vi "configure.vi"(8 "error in (no error)":errorcluster, 10 "SerialConfig":T1={"Serial Protocol"=enum."RS485", "Protocol Parameters"={"VISA resource name"="", "Baud Rate"=9600, "Data Bits"=8, "Parity"=enum."None", "Flow Control"=0, "Stop Bits"=10, "Timeout (ms)"=10000}} {"Protocol Parameters"."Stop Bits" items=["1.0"=10, "1.5"=15, "2.0"=20]; "Protocol Parameters"."Flow Control" items=["None", "XON/XOFF", "RTS/CTS", "XON/XOFF & RTS/CTS", "DTR/DSR", "XON/XOFF & DTR/DSR"]; "Protocol Parameters"."Data Bits" min=5 max=8 step=1}, 11 "SerialCommunicator in":refnum<class "SerialCommunicator.lvclass">) -> (0 "error out":errorcluster, 3 "SerialCommunicator out":refnum<class "SerialCommunicator.lvclass">)   [LabVIEW 2013, in "SerialProtocols.lvlib" / "SerialCommunicator.lvclass"]
uses:
  <userlib>/Common/SerialProtocols/SerialCommunicator/SerialCommunicator.lvclass
  <userlib>/Common/SerialProtocols/Configuration/SerialConfig.ctl
  <userlib>/Common/SerialProtocols/Configuration/SerialProtocol.ctl
  <userlib>/Common/SerialProtocols/Configuration/ProtocolParameters.ctl
  <userlib>/Common/SerialProtocols/SerialCommunicator/SerialCommunicator.lvclass/SerialCommunicator.ctl
  <userlib>/Common/SerialProtocols/SerialProtocolFactory/ISerialProtocolFactory/ISerialProtocolFactory.lvclass
  <userlib>/Common/SerialProtocols/SerialProtocol/SerialProtocol/SerialProtocol.lvclass
  <userlib>/Common/SerialProtocols/SerialProtocols.lvlib
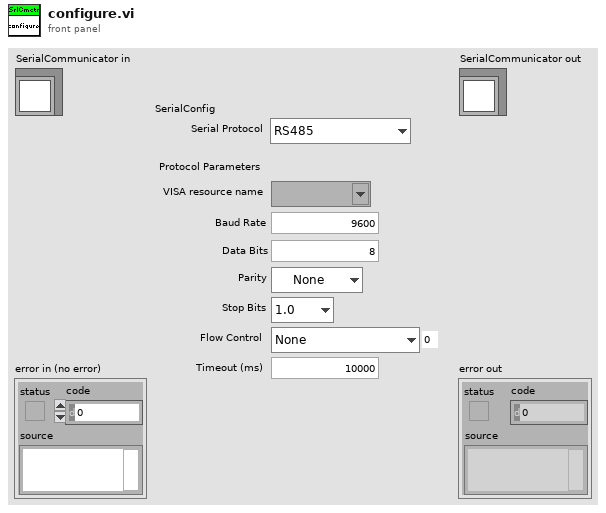
[diagram p1: front panel]
types:
  T1 = typedef "SerialProtocols.lvlib/SerialConfig.ctl" = cluster{"Serial Protocol":T2, "Protocol Parameters":T3}
  T2 = typedef "SerialProtocols.lvlib/SerialProtocol.ctl" = enum16{"RS232", "RS485", "SerialSimulator"}
  T3 = typedef "SerialProtocols.lvlib/ProtocolParameters.ctl" = cluster{"VISA resource name":refnum<visa-resource-name>, "Baud Rate":u32, "Data Bits":u16, "Parity":enum16{"None", "Odd", "Even", "Mark", "Space"}, "Flow Control":u16, "Stop Bits":u16, "Timeout (ms)":u32}
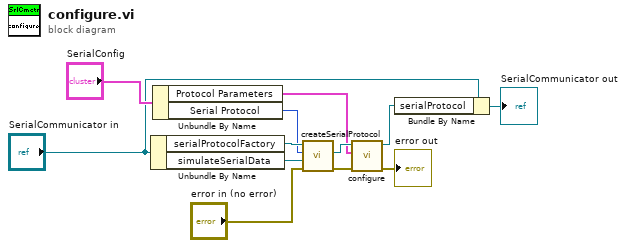
[diagram p0: block diagram]
diagram:
  n1 = Unbundle By Name("SerialCommunicator in") -> ("serialProtocolFactory"=w3:refnum<class "ISerialProtocolFactory.lvclass">, "simulateSerialData"=w1:refnum<class "SimulateSerialData.lvclass">)
  n2 = Unbundle By Name("SerialConfig") -> ("Protocol Parameters"=w9:T3, "Serial Protocol"=w2:T2)
  n3 = call-dynamic "createSerialProtocol.vi"("error in (no error)"="error in (no error)", "simulateSerialData"=w1, "Serial Protocol"=w2, "ISerialCommFactory in"=w3) -> ("error out"=w12:errorcluster, "serialProtocol"=w10:refnum<class "SerialProtocol.lvclass">)  [unwired: 5 in, 1 out]
  n4 = call-dynamic "configure.vi"("error in (no error)"=w12, "Protocol Parameters"=w9, "SerialProtocol in"=w10) -> ("error out"=→"error out":errorcluster, "SerialProtocol out"=w7:refnum<class "SerialProtocol.lvclass">)  [unwired: 7 in]
  n5 = Bundle By Name(cluster="SerialCommunicator in", "serialProtocol"=w7) -> (→"SerialCommunicator out":refnum<class "SerialCommunicator.lvclass">)
